vi "Line Counter.vi"(7 "Action (Increment)":T1=enum."Increment", 8 "error in (no error)":errorcluster, 10 "# of lines to increment (1)":i32=1) -> (0 "error out":errorcluster, 3 "Current Line":i32)   [LabVIEW 2013, in "XML Parser.lvclass"]
uses:
  XML Parser.lvclass
  lineCounter_action.ctl
  XML Parser.lvclass/XML Parser.ctl
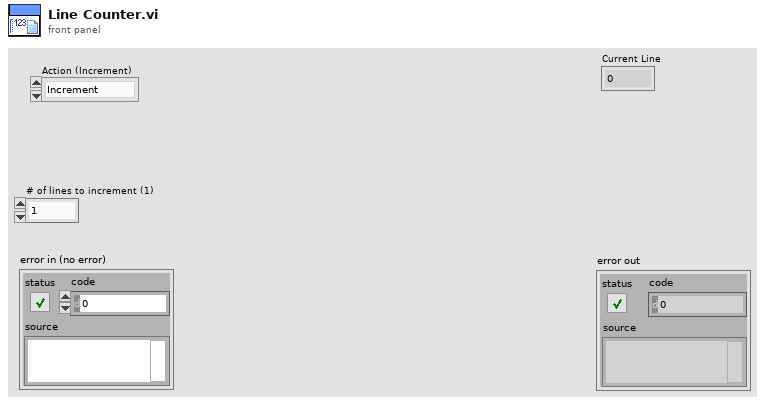
[diagram p1: front panel]
types:
  T1 = typedef "XML Parser.lvclass/lineCounter_action.ctl" = enum16{"Init", "Reset", "Increment", "Get Current Line"}
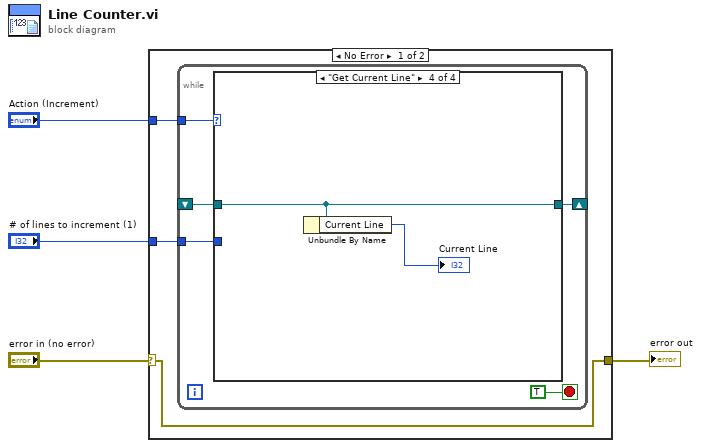
[diagram p0: block diagram]
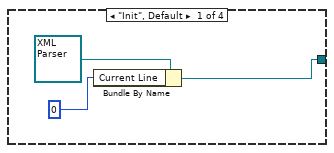
[diagram p2: hidden frame]
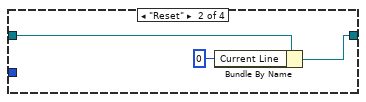
[diagram p3: hidden frame]
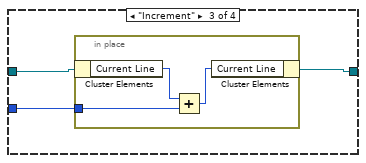
[diagram p4: hidden frame]
diagram:
  n1 = case shown="No Error" "error in (no error)" {
    selector: "error in (no error)" -> [w6 w27]
    tunnel: "Action (Increment)" -> [w7 _]
    tunnel: [w6 w27] -> w2
    tunnel: "# of lines to increment (1)" -> [w5 _]
    frame No Error {
      n2 = while {
        tunnel: w7 -> [w12]
        shift-right: [w10] -> _
        shift-left: _ -> [w9]
        tunnel: w5 -> [w8]
        stop <- TRUE stop-if-true
        n3 = case shown="\"Get Current Line\"" w12 {
          tunnel: [w14 w17 w19 w26] -> w10
          tunnel: w9 -> [_ w18 w21 w26]
          tunnel: w8 -> [_ _ w20 _]
          frame "Init", Default {
            n4 = Bundle By Name(cluster=refnum<class "XML Parser.lvclass"> refnum ("XML Parser.lvclass"), "Current Line"=0) -> (w14:refnum<class "XML Parser.lvclass">)
          }
          frame "Reset" {
            n5 = Bundle By Name(cluster=w18, "Current Line"=0) -> (w17:refnum<class "XML Parser.lvclass">)
          }
          frame "Increment" {
            n6 = in-place {
              in-place-border: w20 -> [w23]
              n7 = in-place-cluster #1(w21) -> ("Current Line"=w24:i32)
              n8 = Add(x=w24, y=w23) -> (x+y=w22:i32)
              n9 = in-place-cluster #1("Current Line"=w22) -> (w19:refnum<class "XML Parser.lvclass">)
            }
          }
          frame "Get Current Line" {
            n10 = Unbundle By Name(w26) -> ("Current Line"=→"Current Line":i32)
          }
        }
      }
    }
    frame Error {
    }
  }
  "error out" <- w2
